vi "experiment control.vi"() -> ()   [LabVIEW 2012] (continued)
              n86 = Concatenate Strings(w240, " End" ("string")) -> (w241:string)
              n87 = Concatenate Strings("Begin " ("string"), w240) -> (w237:string)
              n88 = Concatenate Strings("End " ("string"), w240) -> (w236:string)
            }
            n89 = for {
              tunnel: w218 -> [w235] mode=indexing
              tunnel: [w233] -> w211 mode=indexing
              tunnel: [w230] -> w213 mode=indexing
              n90 = Unbundle By Name(w235) -> ("Name"=w232:string)
              n91 = Concatenate Strings("DAC: " ("string"), w232, " Begin" ("string")) -> (w233:string)
              n92 = Concatenate Strings("DAC " ("string"), w232) -> (w230:string)
            }
            n93 = Interleave 1D Arrays(w223, w222) -> (w221:string[])
            n94 = Interleave 1D Arrays(w217, w216) -> (w212:string[])
            n95 = Build Array (concatenate)(w221, w211, w215) -> (w220:string[])
            n96 = Build Array (concatenate)(w212, w213, w215) -> (w214:string[])
            n97 = Build Cluster Array(w220, w214) -> (w219:cluster{string, string}[])
            n98 = property on="Reference" class="CmbBox"(error in=w226, "Strings And Values[]"=w219) -> (error out=w227:errorcluster)  [unwired: 1 in, 1 out]
          }
          frame "UI: Update State Hierarchy" {
            # "This is added to the queue whenever the DIO64 Tasks is updated. It calculates the cumulative time"
            n99 = property on="Machine State" class="Clust (strict)"(error in=w251) -> (error out=w247:errorcluster, "Controls[]"=w246:refnum<vi>[])  [unwired: 1 in, 1 out]
            n100 = for {
              tunnel: w246 -> [w254] mode=indexing
              shift-right: [w255] -> _
              shift-left: w247 -> [w258]
              tunnel: [w257] -> w248 mode=indexing
              tunnel: [w256] -> w249 mode=indexing
              i -> [w256]
              n101 = property class="Ctl"(reference=w254, error in=w258) -> (error out=w255:errorcluster, "Label.Text"=w257:string)  [unwired: 1 out]
            }
            n102 = property on="State Hierarchy" class="LstBox (strict)"("Item Names"=w248, "Item Symbols"=w249) -> (error out=w252:errorcluster)  [unwired: 2 in, 1 out]
          }
          frame "UI: DIO64 Change Labels" {
            # "This updates the picture labels on the DIO64 Tasks. This is the only way to get vertical text labels."
            n103 = local read "Channel Labels"() -> (w260:T10)
            n104 = Transpose 2D Array(2D array=w260) -> (transposed array=w259:T10)
            n105 = for {
              tunnel: w259 -> [w276] mode=indexing
              tunnel: [w275] -> w261 mode=indexing
              n106 = for {
                tunnel: w276 -> [w287] mode=indexing
                tunnel: [w280] -> w275 mode=indexing
                n107 = Unbundle By Name(w287) -> ("Channel"=w286:string, "Name"=w285:string)
                n108 = Concatenate Strings(w286, "  " ("string"), w285) -> (w283:string)
                n109 = call <vilib>:"Draw Text at Point.vi"("text orientation"=T43."Counterclockwise", "[user-specified font]"=T41 {"Font Name:"="Application", "Size"=10, "Strikeout?"=FALSE, "Italic?"=FALSE, "Underline?"=FALSE, "Outline?"=FALSE, "Shadow?"=FALSE, "Bold?"=TRUE}, "desired font(Application)"=T42."User-specified Font", "text"=w283, "alignment(left, top)"=T44 {"horizontal"=enum."left", "vertical"=enum."bottom"}, "origin"=cluster{"x":i16, "y":i16} {"x"=0, "y"=90}) -> ("new picture"=w280:picture)  [unwired: 4 in, 1 out]
              }
            }
            n110 = Index Array(array=w261, index (row)=0) -> (element=w266:picture[])  [unwired: 1 in]
            n111 = Index Array(array=w261, index (row)=1) -> (element=w267:picture[])  [unwired: 1 in]
            n112 = Index Array(array=w261, index (row)=2) -> (element=w268:picture[])  [unwired: 1 in]
            n113 = Index Array(array=w261, index (row)=3) -> (element=w269:picture[])  [unwired: 1 in]
            n114 = local read "DIO64 Labels:skip"() -> (w270:T5)
            n115 = Bundle By Name(cluster=w270, "Channel 1"=w266, "Channel 2"=w267, "Channel 3"=w268, "Channel 4"=w269) -> (w271:T5)
            n116 = local write "DIO64 Labels:skip"(w271) -> ()
          }
          frame "UI: Chop Labels" {
            # "This updates the picture labels on the DIO64 Tasks. This is the only way to get vertical text labels."
            n117 = local read "Chop Labels"() -> (w289:string[])
            n118 = for {
              tunnel: w289 -> [w295] mode=indexing
              tunnel: [w293] -> w288 mode=indexing
              i -> [w294]
              n119 = call <vilib>:"Draw Text at Point.vi"("text orientation"=T43."Counterclockwise", "[user-specified font]"=T41 {"Font Name:"="Application", "Size"=14, "Strikeout?"=FALSE, "Italic?"=FALSE, "Underline?"=FALSE, "Outline?"=FALSE, "Shadow?"=FALSE, "Bold?"=TRUE}, "desired font(Application)"=T42."User-specified Font", "text"=w295, "alignment(left, top)"=T44 {"horizontal"=enum."left", "vertical"=enum."bottom"}, "origin"=cluster{"x":i16, "y":i16} {"x"=0, "y"=150}) -> ()  [unwired: 4 in, 2 out]
              n120 = Bundle("String"=w295, w294) -> (w293:cluster{"String":string, i32})  [unwired: 1 in]
            }
            n121 = property on="Ring" class="Ring (strict)"("StringsAndValues[]"=w288) -> ()  [unwired: 2 in, 2 out]
            n122 = property on="Ring" class="Ring (strict)"("StringsAndValues[]"=w288) -> ()  [unwired: 2 in, 2 out]
          }
          frame "UI: DAC Update Listing" {
            w307 = "T0"
            # "This updates the picture labels on the DIO64 Tasks. This is the only way to get vertical text labels."
            n123 = local read "DAC Tasks"() -> (w306:T8)
            n124 = for {
              tunnel: w306 -> [w317] mode=indexing
              tunnel: [w316] -> w309 mode=indexing
              n125 = Unbundle By Name(w317) -> ("Name"=w316:string)
            }
            n126 = property on="DAC Listing 2" class="LstBox (strict)"("Item Names"=w309) -> ()  [unwired: 2 in, 2 out]
            n127 = for {
              tunnel: w306 -> [w315] mode=indexing
              tunnel: [w314] -> w305 mode=indexing
              n128 = Unbundle By Name(w315) -> ("Name"=w313:string)
              n129 = Bundle("Name"=w313, "Name"=w313) -> (w314:cluster{"Name":string, "Name":string})  [unwired: 1 in]
            }
            n130 = Bundle(w307, w307) -> (w308:cluster{string, string})  [unwired: 1 in]
            n131 = Build Array (concatenate)(w308, w305) -> (w304:cluster{"Name":string, "Name":string}[])
            n132 = property on="Task" class="CmbBox"(error in=w311, "Strings And Values[]"=w305) -> (error out=w303:errorcluster)  [unwired: 1 in, 1 out]
            n133 = property on="Reference" class="CmbBox"(error in=w303, "Strings And Values[]"=w304) -> (error out=w310:errorcluster)  [unwired: 1 in, 1 out]
            n134 = Enqueue Element At Opposite End(queue=w302, element="UI: Update Scan References") -> ()  [unwired: 2 in, 3 out]
          }
          frame "UI: DAC Update Graph2" {
            # "This updates the picture labels on the DIO64 Tasks. This is the only way to get vertical text labels."
            n135 = property on="DAC Tasks" class="Arr (strict)"() -> ("Index Values"=w323:u32[])  [unwired: 2 in, 2 out]
            n136 = local read "DAC Tasks"() -> (w324:T8)
            n137 = Index Array(array=w323) -> (element=w327:u32)  [unwired: 1 in]
            n138 = Index Array(array=w324, index=w327) -> (element=w326:T55)
            n139 = Unbundle By Name(w326) -> ("DAC"=w325:cluster{"Time":dbl, "Voltage":dbl[]}[])
            n140 = for {
              tunnel: w325 -> [w347] mode=indexing
              tunnel: [w346] -> w321 mode=indexing
              tunnel: [w345] -> w320 mode=indexing
              n141 = Unbundle By Name(w347) -> ("Time"=w346:dbl, "Voltage"=w345:dbl[])
            }
            n142 = Transpose 2D Array(2D array=w320) -> (transposed array=w322:dbl[][])
            n143 = for {
              tunnel: w321 -> [w336]
              tunnel: w322 -> [w337] mode=indexing
              tunnel: [w331] -> w319 mode=indexing
              n144 = Build Cluster Array(w336, w337) -> (w335:cluster{"Time":dbl, "Voltage":dbl}[])
              n145 = Sort 1D Array(array=w335) -> (sorted array=w334:cluster{"Time":dbl, "Voltage":dbl}[])
              n146 = for {
                tunnel: w334 -> [w340] mode=indexing
                tunnel: [w339] -> w333 mode=indexing
                tunnel: [w338] -> w332 mode=indexing
                n147 = Unbundle(w340) -> ("Time"=w338:dbl, "Voltage"=w339:dbl)
              }
              n148 = Bundle(w332, w333) -> (w331:cluster{dbl[], dbl[]})  [unwired: 1 in]
            }
            n149 = flat-sequence {
              tunnel: w319 -> [w341]
              tunnel: [w341] -> w328
              tunnel: w328 -> [w342]
              frame #0 {
                "DAC Waveforms 3" <- w341
              }
              frame #1 {
                n150 = for {
                  tunnel: w342 -> [_] mode=indexing
                  i -> [w344]
                  n151 = property on="DAC Waveforms 3" class="XYGraph (strict)"("Active Plot"=w344, "Plot.Line Width"=u8 3) -> ()  [unwired: 2 in, 2 out]
                }
              }
            }
          }
          frame "UI: Get Case Strings" {
            # "This is very complicated. I don't recommend messing with it. It uses undocumented Labview features, such as scripting.\nIt grabs the names of the cases from this event case and stores them in an array. This way we can tab complete commands, and other things flow together nicely."
            n152 = control-ref of="This VI"() -> (w366:refnum<vi>)
            n153 = property class="VI"(reference=w366, error in=w351) -> (error out=w364:errorcluster, "Diagram"=w363:refnum<vi>)  [unwired: 1 out]
            n154 = property class="TopLvlDiag"(reference=w363, error in=w364) -> (error out=w362:errorcluster, "AllObjs[]"=w365:refnum<vi>[])  [unwired: 1 out]
            n155 = while {
              tunnel: w365 -> [w412] mode=indexing
              tunnel: [w410] -> w367
              stop <- w409 continue-if-true
              w411 = refnum<vi> refnum  # WhileLoop
              n156 = To More Specific Class(target class=w411, reference=w412) -> (specific class reference=w410:refnum<vi>, error out=w409:errorcluster)  [unwired: 1 in]
            }
            n157 = property class="WLoop"(reference=w367, error in=w362) -> (error out=w359:errorcluster, "Diagram.AllObjs[]"=w357:refnum<vi>[])  [unwired: 1 out]
            n158 = while {
              tunnel: w357 -> [w402] mode=indexing
              tunnel: [w400] -> w360
              stop <- w399 continue-if-true
              w401 = refnum<vi> refnum  # Sequence
              n159 = To More Specific Class(target class=w401, reference=w402) -> (specific class reference=w400:refnum<vi>, error out=w399:errorcluster)  [unwired: 1 in]
            }
            n160 = property class="Seq"(reference=w360, error in=w359) -> (error out=w358:errorcluster, "Frames[]"=w353:refnum<vi>[])  [unwired: 1 out]
            n161 = for {
              tunnel: [w392] -> w356
              tunnel: w353 -> [w390] mode=indexing
              shift-right: [w391] -> w355
              shift-left: w358 -> [w394]
              stop <- w389 continue-if-true
              n162 = property class="Diag"(reference=w390, error in=w394) -> (error out=w391:errorcluster, "AllObjs[]"=w393:refnum<vi>[])  [unwired: 1 out]
              n163 = for {
                tunnel: w393 -> [w398] mode=indexing
                tunnel: [w396] -> w392
                tunnel: [w395] -> w389
                stop <- w395 continue-if-true
                w397 = refnum<vi> refnum  # CaseStructure
                n164 = To More Specific Class(target class=w397, reference=w398) -> (specific class reference=w396:refnum<vi>, error out=w395:errorcluster)  [unwired: 1 in]
              }
            }
            n165 = property class="CaseSel"(reference=w356, error in=w355) -> (error out=w348:errorcluster, "FrameNames"=w354:string[])  [unwired: 1 out]
            n166 = for {
              tunnel: w354 -> [w406] mode=indexing
              tunnel: [w403] -> w361 mode=indexing
              n167 = String Length(string=w406) -> (length=w405:i32)
              n168 = Subtract(x=w405, y=4) -> (x-y=w407:i32)
              n169 = String Subset(string=w406, offset (0)=2, length (rest)=w407) -> (substring=w403:string)
            }
            n170 = Array Subset(array=w361, index=6) -> (w349:string[])  [unwired: 1 in]
            n171 = while {
              shift-right: [w375] -> w350
              shift-left: w349 -> [w376]
              stop <- w373 stop-if-true
              n172 = for {
                tunnel: w376 -> [w385] mode=indexing
                tunnel: [w382] -> w374
                tunnel: [w381] -> w373
                i -> [w382]
                stop <- w381 continue-if-true
                n173 = Match Pattern(string=w385, regular expression="^-----") -> (offset past match=w383:i32)  [unwired: 1 in, 3 out]
                n174 = Less Than 0?(x=w383) -> (x < 0?=w381:bool)
              }
              n175 = case shown="False" w373 {
                tunnel: w376 -> [w379 w380]
                tunnel: [w378 w380] -> w375
                tunnel: w374 -> [w377 _]
                frame False {
                  n176 = Delete From Array(array=w379, index=w377) -> (array with subset deleted=w378:string[])  [unwired: 1 in, 1 out]
                }
                frame True {
                }
              }
            }
            n177 = property on="Help Function Names" class="LstBox (strict)"(error in=w348, "Item Names"=w349) -> (error out=w372:errorcluster)  [unwired: 1 in, 1 out]
            n178 = for {
              tunnel: w350 -> [w388] mode=indexing
              tunnel: [w386] -> w368 mode=indexing
              n179 = Bundle(w388, 0) -> (w386:cluster{string, i32})  [unwired: 1 in]
            }
            n180 = local write "debug timing"(w368) -> ()
            n181 = Bundle By Name(cluster=w371, "Command Names"=w350) -> (w370:T52)
          }
          frame "UI: Get Case Documentation" {
            # "This is very complicated. I don't recommend messing with it. It uses undocumented Labview features, such as scripting.\nIt grabs the names of the cases from this event case and stores them in an array. This way we can tab complete commands, and other things flow together nicely."
            n182 = control-ref of="This VI"() -> (w440:refnum<vi>)
            n183 = property class="VI"(reference=w440, error in=w426) -> (error out=w438:errorcluster, "Diagram"=w437:refnum<vi>)  [unwired: 1 out]
            n184 = property class="TopLvlDiag"(reference=w437, error in=w438) -> (error out=w436:errorcluster, "AllObjs[]"=w439:refnum<vi>[])  [unwired: 1 out]
            n185 = while {
              tunnel: w439 -> [w492] mode=indexing
              tunnel: [w490] -> w441
              stop <- w489 continue-if-true
              w491 = refnum<vi> refnum  # WhileLoop
              n186 = To More Specific Class(target class=w491, reference=w492) -> (specific class reference=w490:refnum<vi>, error out=w489:errorcluster)  [unwired: 1 in]
            }
            n187 = property class="WLoop"(reference=w441, error in=w436) -> (error out=w433:errorcluster, "Diagram.AllObjs[]"=w431:refnum<vi>[])  [unwired: 1 out]
            n188 = while {
              tunnel: w431 -> [w482] mode=indexing
              tunnel: [w480] -> w434
              stop <- w479 continue-if-true
              w481 = refnum<vi> refnum  # Sequence
              n189 = To More Specific Class(target class=w481, reference=w482) -> (specific class reference=w480:refnum<vi>, error out=w479:errorcluster)  [unwired: 1 in]
            }
            n190 = property class="Seq"(reference=w434, error in=w433) -> (error out=w432:errorcluster, "Frames[]"=w428:refnum<vi>[])  [unwired: 1 out]
            n191 = for {
              tunnel: [w472] -> w419
              tunnel: w428 -> [w470] mode=indexing
              shift-right: [w471] -> w430
              shift-left: w432 -> [w474]
              stop <- w469 continue-if-true
              n192 = property class="Diag"(reference=w470, error in=w474) -> (error out=w471:errorcluster, "AllObjs[]"=w473:refnum<vi>[])  [unwired: 1 out]
              n193 = for {
                tunnel: w473 -> [w478] mode=indexing
                tunnel: [w476] -> w472
                tunnel: [w475] -> w469
                stop <- w475 continue-if-true
                w477 = refnum<vi> refnum  # CaseStructure
                n194 = To More Specific Class(target class=w477, reference=w478) -> (specific class reference=w476:refnum<vi>, error out=w475:errorcluster)  [unwired: 1 in]
              }
            }
            n195 = property class="CaseSel"(reference=w419, error in=w430) -> (error out=w420:errorcluster, "FrameNames"=w429:string[])  [unwired: 1 out]
            n196 = property class="CaseSel"(reference=w419, error in=w420) -> (error out=w422:errorcluster, "Frames[]"=w425:refnum<vi>[])  [unwired: 1 out]
            n197 = for {
              tunnel: w425 -> [w462] mode=indexing
              tunnel: [w455] -> w423 mode=indexing
              tunnel: w422 -> [w457]
              tunnel: [w457] -> w421 mode=indexing
              n198 = property class="Diag"(reference=w462, error in=w457) -> (error out=w459:errorcluster, "AllObjs[]"=w461:refnum<vi>[])  [unwired: 1 out]
              n199 = for {
                tunnel: w461 -> [w468] mode=indexing
                tunnel: [w466] -> w460
                tunnel: [w465] -> w458
                tunnel: w459 -> [w464]
                stop <- w465 continue-if-true
                w467 = refnum<vi> refnum  # Text
                n200 = To More Specific Class(target class=w467, reference=w468, error in=w464) -> (specific class reference=w466:refnum<vi>, error out=w465:errorcluster)
              }
              n201 = property class="Txt"(reference=w460, error in=w458) -> (error out=w456:errorcluster, "Text"=w454:string)  [unwired: 1 out]
              n202 = case shown="Error" w456 {
                tunnel: [w463 _] -> w455
                tunnel: w454 -> [w463 _]
                frame No Error {
                }
                frame Error {
                }
              }
            }
            n203 = for {
              tunnel: w429 -> [w486] mode=indexing
              tunnel: [w483] -> w435 mode=indexing
              n204 = String Length(string=w486) -> (length=w485:i32)
              n205 = Subtract(x=w485, y=4) -> (x-y=w487:i32)
              n206 = String Subset(string=w486, offset (0)=2, length (rest)=w487) -> (substring=w483:string)
            }
            n207 = Merge Errors(w421) -> (w417:errorcluster)
            n208 = Array Subset(array=w435, index=6) -> (w414:string[])  [unwired: 1 in]
            n209 = Array Subset(array=w423, index=6) -> (w415:string[])  [unwired: 1 in]
            n210 = for {
              shift-right: [w444] -> w413
              shift-left: string[] [] -> [w445]
              tunnel: w414 -> [w446] mode=indexing
              tunnel: w415 -> [w447] mode=indexing
              n211 = Match Pattern(string=w446, regular expression="^-----") -> (offset past match=w448:i32)  [unwired: 1 in, 3 out]
              n212 = Less Than 0?(x=w448) -> (x < 0?=w443:bool)
              n213 = case shown="True" w443 {
                tunnel: w447 -> [_ w453]
                tunnel: w445 -> [w450 w452]
                tunnel: [w450 w451] -> w444
                frame False {
                }
                frame True {
                  n214 = Build Array (concatenate)(w452, w453) -> (w451:string[])
                }
              }
            }
            "documentation" <- w413
          }
          frame "---------- Macro ----------" {
            # "Do not put any code in this frame.\n(It is a separator no-op. You can make a copy of this frame to create a new Macro frame)"
          }
          frame "Macro: Initialize" {
            # "Initialization Macro\n(This is called once, when the VI starts)"
            n215 = case shown="False" "test" {
              tunnel: [w515 "Clear\nData: Initialize\nInitialize Core Data\nUI: Initialize\nUI: Front Panel State >> Open\nUI: Get Case Strings\nUI: DIO64 Update Control\nUI: DIO64 Change Labels\n# UI: DIO64 Update Listing\nUI: DAC Update Listing\n# This is some fun text for the UI.\nDebug: Console >> ****************************\nDebug: Console >> **  Starting Experiment Control  **\nDebug: Console >> ****************************\n#Now start up the hardware\nWavemeter: Initialise\nWavemeter: Start\nScope: Initialise >> TDS5034B\nScope: Initialise >> TDS2014\nDIO64: Initialise\nDAC: Clear\nLaser: Initialize DAC\nDDS: Set Clock\nDDS: Set Frequency >> 1\nDDS: Set Frequency >> 2\nDDS: Set Frequency >> 3\nDDS: Set Frequency >> 4\nTrap DDS: Set Clock\nTrap DDS: Connect Serial\nQuadDVM: Initialize\nMagnetometer: Initialize\nCoils: Initialize\nUSB DAQ: Initialize\nTrap Agilent: Initialize\nTrap Agilent: Set\nDepletion Agilent: Initialize\nDepletion Agilent: Set\nGo Today\nSwitch: Set Machine State\nChillax: Initialize"] -> w500
              frame True {
                w515 = "Clear\nData: Initialize\nInitialize Core Data\nUI: Initialize\nUI: Front Panel State >> Open\nUI: Get Case Strings\nUI: DIO64 Update Control\nUI: DIO64 Change Labels\nUI: DAC Update Listing\n# This is some fun text for the UI.\nDebug: Console >> ****************************\nDebug: Console >> **  Starting Experiment Control  **\nDebug: Console >> ****************************\n#Now start up the hardware\n#Wavemeter: Initialise\n#Wavemeter: Start\n#Scope: Initialise >> TDS5034B\n#Scope: Initialise >> TDS2014\n#DIO64: Initialise\n#DDG: Initialise\n#DAC: Clear\n#DDS: Set Clock\n#DDS: Set Frequency >> 1\n#DDS: Set Frequency >> 2\n#DDS: Set Frequency >> 3\n#DDS: Set Frequency >> 4\n#Trap DDS: Set Clock\n#Trap DDS: Connect Serial\n#Macro: Clear Wavelengths\n#SIM970: Initialize\n"  # Clear Data: Initialize Initialize Core Data UI: Initialize UI: Front Panel State >> Open UI: Get Case Strings UI: DIO64 Update Control UI: DIO64 Change Labels UI: DAC Update Listing # This is some fun text for the UI. Debug: Console >> **************************** Debug: Console >> **  Starting Experiment Control  ** Debug: Console >> **************************** #Now start up the hardware #Wavemeter: Initialise #Wavemeter: Start #Scope: Initialise >> TDS5034B #Scope: Initialise >> TDS2014 #DIO64: Initialise #DDG: Initialise #DAC: Clear #DDS: Set Clock #DDS: Set Frequency >> 1 #DDS: Set Frequency >> 2 #DDS: Set Frequency >> 3 #DDS: Set Frequency >> 4 #Trap DDS: Set Clock #Trap DDS: Connect Serial #Macro: Clear Wavelengths #SIM970: Initialize
              }
              frame False {
              }
            }
            n216 = while {
              shift-right: [w512] -> _
              shift-left: w500 -> [w514]
              tunnel: [w511] -> w501 mode=indexing
              stop <- w509 stop-if-true
              n217 = Match Pattern(string=w514, regular expression="[\\n\\r]+") -> (before substring=w511:string, after substring=w512:string, offset past match=w510:i32)  [unwired: 1 in, 1 out]
              n218 = Less Than 0?(x=w510) -> (x < 0?=w509:bool)
            }
            n219 = Reverse 1D Array(array=w501) -> (reversed array=w499:string[])
            n220 = for {
              tunnel: [w508] -> _
              tunnel: w498 -> [w507]
              shift-right: [w505] -> w496
              shift-left: w497 -> [w506]
              tunnel: w499 -> [w504] mode=indexing
              n221 = Enqueue Element At Opposite End(queue=w507, element=w504, error in (no error)=w506) -> (queue out=w508:refnum<queue>, error out=w505:errorcluster)  [unwired: 1 in, 1 out]
            }
          }
          frame "Macro: Read Wavelengths" {
            # "Initialization Macro\n(This is called once, when the VI starts)"
            n222 = call "string_to_array.vi"("string"="#Wavemeter: Read\nLaser: Read Wavelength >> Stella\nLaser: Read Wavelength >> Jessica\nLaser: Read Wavelength >> Toptica\nLaser: Read Wavelength >> Cora") -> ("array"=w522:string[])
            n223 = call "queue_array_front.vi"("error in"=w517, "array"=w522, "queue in"=w520) -> ("error out"=w518:errorcluster, "queue out"=w519:refnum<queue>)  [unwired: 7 in]
          }
          frame "Macro: Exit" {
            # "Exit Macro\n(This is called once, when the VI exits)"
            n224 = Unbundle By Name(w541) -> ("Core.Close Panel on Exit?"=w540:bool)
            n225 = local read "test"() -> (w534:bool)
            n226 = case shown="False" w534 {
              tunnel: ["# This is some fun text for the UI.\nDebug: Console >> ****************************\nDebug: Console >> **  Exiting Experiment Control  **\nDebug: Console >> ****************************\n#\nData: Cleanup\n#Scope: Close >> TDS5034B\n#Scope: Close >> TDS2014\n#DIO64: Close\n#DDG: Close\n#Wavemeter: Stop\n#Wavemeter: Close\n#SIM970: Close\n#Trap DDS: Connect Serial\nExit" "# This is some fun text for the UI.\nDebug: Console >> ****************************\nDebug: Console >> **  Exiting Experiment Control  **\nDebug: Console >> ****************************\n#\nData: Cleanup\nScope: Close >> TDS5034B\nScope: Close >> TDS2014\nDIO64: Close\nWavemeter: Stop\nWavemeter: Close\nQuadDVM: Close\nTrap DDS: Connect Serial\nMagnetometer: Close\nCoils: Close\nTrap Agilent: Close\nDepletion Agilent: Close\nLaser: Close DAC\nChillax: Close\nExit"] -> w536
              frame True {
              }
              frame False {
              }
            }
            n227 = property on="Input" class="TabCtl (strict)"() -> ("Pages"=w526:refnum<vi>[])  [unwired: 2 in, 2 out]
            n228 = property on="Output" class="TabCtl (strict)"() -> ("Pages"=w525:refnum<vi>[])  [unwired: 2 in, 2 out]
            n229 = Select(t="UI: Front Panel State >> Close", s=w540, f="") -> (s? t:f=w537:string)
            n230 = Build Array (concatenate)(w526, w525) -> (w524:refnum<vi>[])
            n231 = for {
              tunnel: w524 -> [w543] mode=indexing
              n232 = property class="Page"(reference=w543, "PageVis"=TRUE ("Page Visible")) -> ()  [unwired: 1 in, 2 out]
            }
            n233 = call <vilib>:"Add State(s) to Queue__jki_lib_state_machine.vi"("State(s) in (\"\")"=w537, "State(s) at Back (\"\")"=w536) -> ("States Out"=w530:string)  [unwired: 13 in]
            n234 = while {
              shift-right: [w552] -> _
              shift-left: w530 -> [w554]
              tunnel: [w551] -> w533 mode=indexing
              stop <- w549 stop-if-true
              n235 = Match Pattern(string=w554, regular expression="[\\n\\r]+") -> (before substring=w551:string, after substring=w552:string, offset past match=w550:i32)  [unwired: 1 in, 1 out]
              n236 = Less Than 0?(x=w550) -> (x < 0?=w549:bool)
            }
            n237 = property on="test" class="Bool (strict)"("DisabledEnum"=T39."Enabled" ("Disabled")) -> ()  [unwired: 2 in, 2 out]
            n238 = Reverse 1D Array(array=w533) -> (reversed array=w532:string[])
            n239 = for {
              tunnel: [w548] -> w527
              tunnel: w531 -> [w547]
              shift-right: [w545] -> w528
              shift-left: w529 -> [w546]
              tunnel: w532 -> [w544] mode=indexing
              n240 = Enqueue Element At Opposite End(queue=w547, element=w544, error in (no error)=w546) -> (queue out=w548:refnum<queue>, error out=w545:errorcluster)  [unwired: 1 in, 1 out]
            }
          }
          frame "---------- Reserved ----------" {
            # "Template Separator\n(You can make a copy of, or modify, this frame)"
          }
          frame "Function" {
            # "This command calls the custom functions specified in the programming tab"
            n241 = local read "Functions"() -> (w568:cluster{"Name":string, "Body":string}[])
            n242 = for {
              tunnel: w568 -> [w590] mode=indexing
              tunnel: [w589] -> w566 mode=indexing
              tunnel: [w588] -> w567 mode=indexing
              n243 = Unbundle By Name(w590) -> ("Body"=w589:string, "Name"=w588:string)
            }
            n244 = Search 1D Array(1D array=w567, element=w569) -> (index of element=w565:i32)  [unwired: 1 in]
            n245 = Index Array(array=w566, index=w565) -> (element=w563:string)
            n246 = Greater Or Equal To 0?(x=w565) -> (x >= 0?=w564:bool)
            n247 = case shown="True" w564 {
              tunnel: w563 -> [_ w575]
              tunnel: w562 -> [w571 w574]
              tunnel: [w571 w573] -> w561
              tunnel: w560 -> [_ w572]
              frame False {
              }
              frame True {
                n248 = while {
                  shift-right: [w585] -> _
                  shift-left: w575 -> [w587]
                  tunnel: [w584] -> w576 mode=indexing
                  stop <- w582 stop-if-true
                  n249 = Match Pattern(string=w587, regular expression="[\\n\\r]+") -> (before substring=w584:string, after substring=w585:string, offset past match=w583:i32)  [unwired: 1 in, 1 out]
                  n250 = Less Than 0?(x=w583) -> (x < 0?=w582:bool)
                }
                n251 = Reverse 1D Array(array=w576) -> (reversed array=w577:string[])
                n252 = for {
                  tunnel: w577 -> [w581] mode=indexing
                  shift-right: [w579] -> w573
                  shift-left: w574 -> [w580]
                  tunnel: w572 -> [w578]
                  n253 = Enqueue Element At Opposite End(queue=w578, element=w581, error in (no error)=w580) -> (error out=w579:errorcluster)  [unwired: 1 in, 2 out]
                }
              }
            }
          }
          frame "Clear" {
            # "This command calls the custom functions specified in the programming tab"
            n254 = local write "stdout"("" ("Remaining States")) -> ()
          }
          frame "Abort" {
            # "This command calls the custom functions specified in the programming tab"
            n255 = Flush Queue(queue=w597, error in (no error)=w596) -> (queue out=w598:refnum<queue>, error out=w595:errorcluster)  [unwired: 1 out]
          }
          frame "Test" {
            # "This command calls the custom functions specified in the programming tab"
            n256 = case shown="True" "Test" {
              tunnel: w604 -> [w607 w613]
              tunnel: [w607 w612] -> w602
              tunnel: [w606 w611] -> w600
              tunnel: w601 -> [w606 w608]
              frame False {
              }
              frame True {
                n257 = while {
                  tunnel: "[\\n\\r]+" ("regular expression") -> [w625]
                  shift-right: [w624] -> _
                  shift-left: "Test Commands" -> [w626]
                  tunnel: [w623] -> w610 mode=indexing
                  stop <- w621 stop-if-true
                  n258 = Match Pattern(string=w626, regular expression=w625) -> (before substring=w623:string, after substring=w624:string, offset past match=w622:i32)  [unwired: 1 in, 1 out]
                  n259 = Less Than 0?(x=w622) -> (x < 0?=w621:bool)
                }
                n260 = Reverse 1D Array(array=w610) -> (reversed array=w614:string[])
                n261 = for {
                  tunnel: w614 -> [w618] mode=indexing
                  shift-right: [w619] -> w612
                  shift-left: w613 -> [w620]
                  shift-right: [w616] -> w611
                  shift-left: w608 -> [w617]
                  n262 = Enqueue Element At Opposite End(queue=w620, element=w618, error in (no error)=w617) -> (queue out=w619:refnum<queue>, error out=w616:errorcluster)  [unwired: 1 in, 1 out]
                }
              }
            }
          }
          frame "Pause" {
            # "This pauses the experiment"
            n263 = Unbundle By Name(w628) -> ("Paused"=w627:bool)
            n264 = case shown="False" w627 {
              tunnel: w628 -> [w649 w652]
              tunnel: [w648 w652] -> w633
              tunnel: w632 -> [w647 w651]
              tunnel: w631 -> [w646 w650]
              tunnel: [w641 w651] -> w630
              tunnel: [w639 w650] -> w629
              frame False {
                w634 = TRUE ("Pause")
                n265 = Flush Queue(queue=w647, error in (no error)=w646) -> (queue out=w642:refnum<queue>, remaining elements=w645:string[], error out=w640:errorcluster)
                n266 = call <vilib>:"Application Directory.vi"() -> ("Application Directory"=w644:path)
                n267 = local write "pause:skip"(w634) -> ()
                n268 = Bundle By Name(cluster=w649, "Paused Queue"=w645, "Paused"=w634) -> (w648:T52)
                n269 = Build Path(base path=w644, name or relative path="pause_state.ubin") -> (appended path=w635:path)
                n270 = Path To String(path=w635) -> (string=w636:string)
                n271 = Concatenate Strings("uBinary: Save >> " ("name or relative path"), w636) -> (w637:string)
                n272 = Enqueue Element At Opposite End(queue=w642, element=w637, error in (no error)=w640) -> (queue out=w641:refnum<queue>, error out=w639:errorcluster)  [unwired: 1 in, 1 out]
              }
              frame True {
              }
            }
          }
          frame "Unpause" {
            # "This unpauses the experiment"
            n273 = Unbundle By Name(w654) -> ("Paused Queue"=w655:string[], "Paused"=w656:bool)
            n274 = case shown="True" w656 {
              tunnel: w660 -> [w663 w682]
              tunnel: w659 -> [w662 w681]
              tunnel: [w662 w673] -> w658
              tunnel: [w663 w672] -> w657
              tunnel: w655 -> [_ w671]
              tunnel: w654 -> [w661 w670]
              tunnel: [w661 w669] -> w653
              frame False {
              }
              frame True {
                n275 = call "queue_array_front.vi"("error in"=w681, "array"=w671, "queue in"=w682) -> ("error out"=w674:errorcluster, "queue out"=w666:refnum<queue>)  [unwired: 7 in]
                n276 = call <vilib>:"Application Directory.vi"() -> ("Application Directory"=w680:path)
                n277 = call "queue_array_front.vi"("array"=string[] ["Scope: Settings >> TDS5034B", "Scope: Trigger Settings >> TDS5034B"], "queue in"=w666) -> ("queue out"=w665:refnum<queue>)  [unwired: 8 in, 1 out]
                n278 = Build Path(base path=w680, name or relative path="pause_state.ubin") -> (appended path=w676:path)
                n279 = Path To String(path=w676) -> (string=w677:string)
                n280 = Concatenate Strings("uBinary: Load >> , " ("name or relative path"), w677) -> (w675:string)
                n281 = Enqueue Element At Opposite End(queue=w665, element=w675, error in (no error)=w674) -> (queue out=w672:refnum<queue>, error out=w673:errorcluster)  [unwired: 1 in, 1 out]
                n282 = Bundle By Name(cluster=w670, "Paused Queue"=string[] [], "Paused"=FALSE) -> (w669:T52)
              }
            }
          }
          frame "Wait" {
            # "This command calls the custom functions specified in the programming tab"
            n283 = Index Array(array=w684) -> (element=w683:string)  [unwired: 1 in]
            n284 = Decimal String To Number(string=w683) -> (number=w686:i32)  [unwired: 2 in, 1 out]
            n285 = Wait (ms)(milliseconds to wait=w686) -> ()  [unwired: 1 out]
          }
          frame "Sync" {
            # "This command calls the custom functions specified in the programming tab"
            n286 = call <vilib>:"Create Rendezvous.vi"("error in (no error)"=w690, "name (unnamed)"="sync") -> ("error out"=w693:errorcluster, "rendezvous"=w694:T56)  [unwired: 3 in, 1 out]
            n287 = call <vilib>:"Wait at Rendezvous.vi"("error in (no error)"=w693, "rendezvous"=w694) -> ("error out"=w691:errorcluster, "rendezvous out"=w692:T56)  [unwired: 3 in, 1 out]
            n288 = call <vilib>:"Destroy Rendezvous.vi"("error in (no error)"=w691, "rendezvous"=w692) -> ("error out"=w689:errorcluster)  [unwired: 4 in, 1 out]
          }
          frame "Tick" {
            # "This command calls the custom functions specified in the programming tab"
            n289 = Tick Count (ms)() -> (millisecond timer value=w699:u32)
            n290 = Bundle By Name(cluster=w701, "Time"=w699) -> (w700:T52)
          }
          frame "Tock" {
            # "This command calls the custom functions specified in the programming tab"
            n291 = Unbundle By Name(w712) -> ("Time"=w711:u32)
            n292 = Tick Count (ms)() -> (millisecond timer value=w710:u32)
            n293 = Subtract(x=w710, y=w711) -> (x-y=w709:u32)
            n294 = Number To Decimal String(number=w709) -> (decimal integer string=w708:string)  [unwired: 1 in]
            n295 = Concatenate Strings("Debug: Console >> " ("string"), w708) -> (w705:string)
            n296 = Enqueue Element(queue=w706, element=w705, error in (no error)=w704) -> (error out=w703:errorcluster)  [unwired: 1 in, 2 out]
          }
          frame "For Loop" {
            # "This command calls the custom functions specified in the programming tab"
            n297 = Flush Queue(queue=w718) -> (remaining elements=w720:string[])  [unwired: 1 in, 2 out]
            n298 = for {
              shift-right: [w752] -> _
              shift-left: 1 -> [w746]
              tunnel: w720 -> [w743] mode=indexing
              tunnel: [w742] -> w722
              tunnel: [w741] -> w721
              i -> [w742]
              stop <- w741 stop-if-true
              n299 = Match Pattern(string=w743, regular expression="#") -> (before substring=w744:string)  [unwired: 1 in, 3 out]
              n300 = Search/Split String(string=w744, search string/char (-)="For Loop" ("search string")) -> (offset of match=w758:i32)  [unwired: 1 in, 2 out]
              n301 = Search/Split String(string=w744, search string/char (-)="While Loop" ("search string")) -> (offset of match=w751:i32)  [unwired: 1 in, 2 out]
              n302 = Search/Split String(string=w744, search string/char (-)="End Loop" ("search string")) -> (offset of match=w757:i32)  [unwired: 1 in, 2 out]
              n303 = Greater Or Equal To 0?(x=w758) -> (x >= 0?=w748:bool)
              n304 = Greater Or Equal To 0?(x=w751) -> (x >= 0?=w749:bool)
              n305 = Greater Or Equal To 0?(x=w757) -> (x >= 0?=w754:bool)
              n306 = Or(x=w748, y=w749) -> (x .or. y?=w747:bool)
              n307 = Increment(x=w746) -> (x+1=w756:i32)
              n308 = Select(t=w756, s=w747, f=w746) -> (s? t:f=w753:i32)
              n309 = Decrement(x=w753) -> (x-1=w755:i32)
              n310 = Select(t=w755, s=w754, f=w753) -> (s? t:f=w752:i32)
              n311 = Equal To 0?(x=w752) -> (x = 0?=w741:bool)
            }
            n312 = Decimal String To Number(string=w719) -> (number=w713:i32)  [unwired: 2 in, 1 out]
            n313 = case shown="True" w721 {
              tunnel: w720 -> [w729 w737]
              tunnel: w722 -> [_ w736]
              tunnel: [w729 w731] -> w714
              tunnel: w713 -> [_ w730]
              frame False {
              }
              frame True {
                n314 = Split 1D Array(array=w737, index=w736) -> (first subarray=w733:string[], second subarray=w734:string[])
                n315 = Array Subset(array=w734, index=1) -> (w732:string[])  [unwired: 1 in]
                n316 = for {
                  N: w730 -> [_]
                  tunnel: w733 -> [w738]
                  shift-right: [w739] -> w731
                  shift-left: w732 -> [w740]
                  n317 = Build Array (concatenate)(w738, w740) -> (w739:string[])
                }
              }
            }
            n318 = Reverse 1D Array(array=w714) -> (reversed array=w717:string[])
            n319 = for {
              tunnel: w718 -> [w728]
              tunnel: w717 -> [w727] mode=indexing
              shift-right: [w725] -> w715
              shift-left: w716 -> [w726]
              n320 = Enqueue Element At Opposite End(queue=w728, element=w727, error in (no error)=w726) -> (error out=w725:errorcluster)  [unwired: 1 in, 2 out]
            }
          }
          frame "While Loop" {
            # "This command calls the custom functions specified in the programming tab"
            n321 = Flush Queue(queue=w769) -> (remaining elements=w762:string[])  [unwired: 1 in, 2 out]
            n322 = for {
              shift-right: [w873] -> _
              shift-left: 1 -> [w867]
              tunnel: w762 -> [w864] mode=indexing
              tunnel: [w863] -> w771
              tunnel: [w862] -> w770
              i -> [w863]
              stop <- w862 stop-if-true
              n323 = Match Pattern(string=w864, regular expression="#") -> (before substring=w865:string)  [unwired: 1 in, 3 out]
              n324 = Search/Split String(string=w865, search string/char (-)="For Loop" ("search string")) -> (offset of match=w879:i32)  [unwired: 1 in, 2 out]
              n325 = Search/Split String(string=w865, search string/char (-)="While Loop" ("search string")) -> (offset of match=w872:i32)  [unwired: 1 in, 2 out]
              n326 = Search/Split String(string=w865, search string/char (-)="End Loop" ("search string")) -> (offset of match=w878:i32)  [unwired: 1 in, 2 out]
              n327 = Greater Or Equal To 0?(x=w879) -> (x >= 0?=w869:bool)
              n328 = Greater Or Equal To 0?(x=w872) -> (x >= 0?=w870:bool)
              n329 = Greater Or Equal To 0?(x=w878) -> (x >= 0?=w875:bool)
              n330 = Or(x=w869, y=w870) -> (x .or. y?=w868:bool)
              n331 = Increment(x=w867) -> (x+1=w877:i32)
              n332 = Select(t=w877, s=w868, f=w867) -> (s? t:f=w874:i32)
              n333 = Decrement(x=w874) -> (x-1=w876:i32)
              n334 = Select(t=w876, s=w875, f=w874) -> (s? t:f=w873:i32)
              n335 = Equal To 0?(x=w873) -> (x = 0?=w862:bool)
            }
            n336 = Concatenate Strings("While Loop >> " ("search string"), w763) -> (w761:string)
            n337 = case shown="True" w770 {
              tunnel: w762 -> [w778 w780]
              tunnel: w771 -> [_ w790]
              tunnel: [w778 w784] -> w765
              tunnel: w763 -> [_ w786]
              tunnel: w761 -> [_ w779]
              frame False {
              }
              frame True {
                n338 = Split 1D Array(array=w780, index=w790) -> (first subarray=w785:string[], second subarray=w782:string[])
                n339 = Match Pattern(string=w786, regular expression=" ") -> (before substring=w788:string, after substring=w789:string)  [unwired: 1 in, 2 out]
                n340 = Build Array (concatenate)(w779, w780) -> (w781:string[])
                n341 = case shown="\"Stella\"" w788 {
                  tunnel: [FALSE w796 w805 w814 w823 w832 w842 w861] -> w783
                  tunnel: w789 -> [_ _ _ _ _ _ w841 _]
                  frame Default {
                  }
                  frame "Stella" {
                    n342 = local read "Stella"() -> (w797:T20)
                    n343 = Unbundle By Name(w797) -> ("scan start"=w804:dbl, "setpoint"=w800:dbl, "scan end"=w803:dbl)
                    n344 = Max & Min(x=w804, y=w803) -> (max(x,y)=w801:dbl, min(x,y)=w802:dbl)
                    n345 = Greater?(x=w801, y=w800) -> (0:w799:bool)
                    n346 = Greater?(x=w800, y=w802) -> (0:w798:bool)
                    n347 = And(x=w799, y=w798) -> (x .and. y?=w796:bool)
                  }
                  frame "Jessica" {
                    n348 = local read "Jessica"() -> (w806:T17)
                    n349 = Unbundle By Name(w806) -> ("scan start"=w813:dbl, "setpoint"=w809:dbl, "scan end"=w812:dbl)
                    n350 = Max & Min(x=w813, y=w812) -> (max(x,y)=w810:dbl, min(x,y)=w811:dbl)
                    n351 = Greater?(x=w810, y=w809) -> (0:w808:bool)
                    n352 = Greater?(x=w809, y=w811) -> (0:w807:bool)
                    n353 = And(x=w808, y=w807) -> (x .and. y?=w805:bool)
                  }
                  frame "Bertha" {
                    n354 = local read "Bertha"() -> (w815:T22)
                    n355 = Unbundle By Name(w815) -> ("scan start"=w822:dbl, "setpoint"=w818:dbl, "scan end"=w821:dbl)
                    n356 = Max & Min(x=w822, y=w821) -> (max(x,y)=w819:dbl, min(x,y)=w820:dbl)
                    n357 = Greater Or Equal?(x=w819, y=w818) -> (x >= y?=w817:bool)
                    n358 = Greater?(x=w818, y=w820) -> (0:w816:bool)
                    n359 = And(x=w817, y=w816) -> (x .and. y?=w814:bool)
                  }
                  frame "Cora" {
                    n360 = local read "Cora"() -> (w824:T21)
                    n361 = Unbundle By Name(w824) -> ("scan start"=w831:dbl, "setpoint"=w827:dbl, "scan end"=w830:dbl)
                    n362 = Max & Min(x=w831, y=w830) -> (max(x,y)=w828:dbl, min(x,y)=w829:dbl)
